vi "Open.vi"(8 "error in":errorcluster, 11 "Standard Engine in":refnum<class "Standard Engine Runtime.lvclass">) -> (0 "error out":errorcluster, 3 "Standard Engine out":refnum<class "Standard Engine Runtime.lvclass">)   [LabVIEW 2013, in "Standard Engine Runtime.lvclass"]
doc: "This VI launches an engine background process that then waits for commands from the other API functions."
uses:
  Standard Engine Runtime.lvclass
  Commands.ctl
  Engine Config Data.ctl
  Configuration/Standard Engine Configuration.lvclass
  <vilib>/NI/Tag Bus Module Framework/runtime/TBM module execution interface.lvclass
  <vilib>/NI/Tag Bus Module Framework/module configuration/TBM module configuration.lvclass
  <vilib>/NI/Module Execution Interface/Engine Runtime/Execution States.ctl
  Engine Process Init Data.ctl
  Standard Engine Runtime.lvclass/Standard Engine Runtime.ctl
  <vilib>/NI/Module Execution Interface/Engine Runtime/Engine Runtime Interface.lvclass
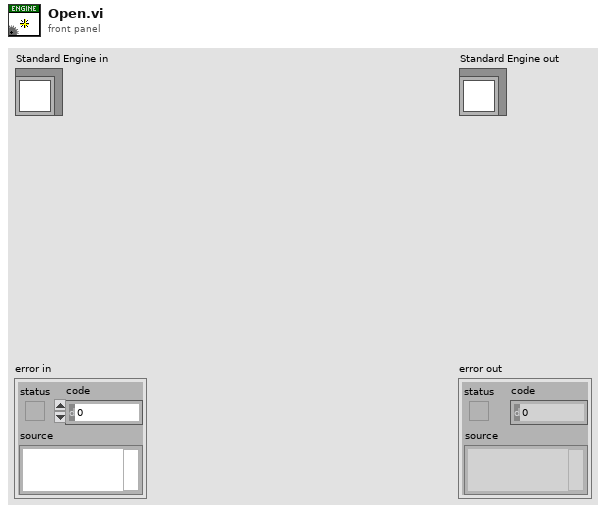
[diagram p1: front panel]
types:
  T1 = typedef "Engine Runtime Interface.lvclass/Execution States.ctl" = enum16{"Initializing", "Paused (Initialized)", "Running", "Set Safe Outputs", "Uninitializing", "Stopped (Uninitialized)", "Error (Uninitialized)", "Safe State (Uninitialized)", "Closed"}
  T2 = typedef "Standard Engine Runtime.lvclass/Engine Process Init Data.ctl" = cluster{"Messages FIFO":refnum<k33>, "Engine Config. Ref":refnum<data-value>, "Status Notifier":refnum<notifier>, "Error Queue":refnum<queue>}
  T3 = typedef "Standard Engine Runtime.lvclass/Engine Config Data.ctl" = cluster{"Engine Configuration":refnum<class "Standard Engine Configuration.lvclass">, "Modules":refnum<class "TBM module execution interface.lvclass">[], "Module Configurations":refnum<class "TBM module configuration.lvclass">[]}
  T4 = typedef "Standard Engine Runtime.lvclass/Commands.ctl" = enum16{"Initialize", "Start", "Pause", "Safe State", "Normal", "Stop", "Shutdown"}
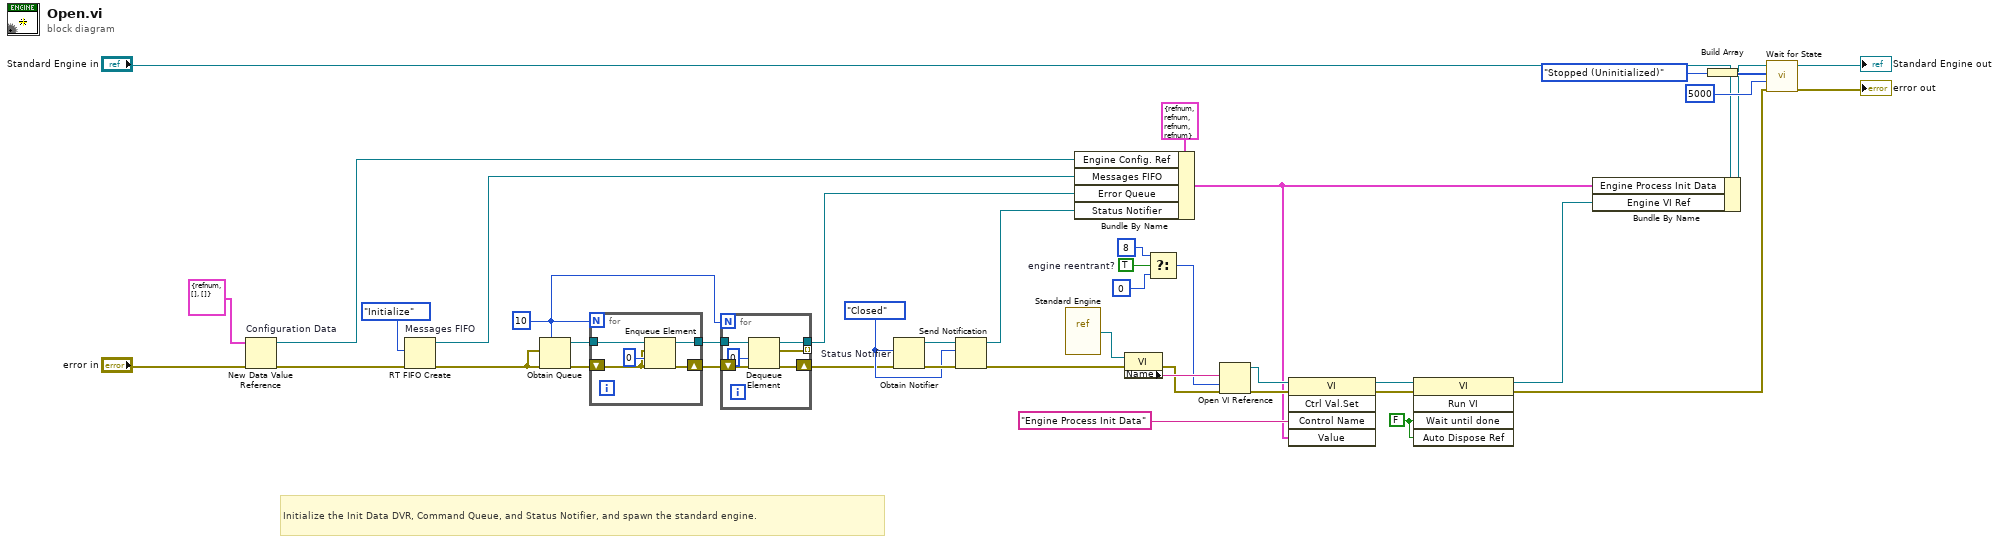
[diagram p0: block diagram]
diagram:
  w1 = FALSE ("Wait Until Done")
  w13 = TRUE  # engine reentrant?
  w23 = 10 ("max queue size (-1, unlimited)")
  w34 = Execution_States."Closed" ("States")
  # "Initialize the Init Data DVR, Command Queue, and Status Notifier, and spawn the standard engine."
  n1 = New Data Value Reference "Configuration Data"(data value=T3 {"Engine Configuration"=refnum, "Modules"=[], "Module Configurations"=[]} ("Engine Configuration Data"), error in="error in") -> (data value reference=w32:refnum<data-value>, error out=w38:errorcluster)
  n2 = RT FIFO Create "Messages FIFO"(1:Commands."Initialize" ("Commands"), 3:w38) -> (8:w31:refnum<k33>, 11:w18:errorcluster)  [unwired: 6 in, 1 out]
  n3 = Obtain Queue(max queue size (-1, unlimited)=w23, element data type=w18, error in (no error)=w18) -> (queue out=w25:refnum<queue>, error out=w24:errorcluster)  [unwired: 2 in, 1 out]
  n4 = for {
    N: w23 -> [_]
    tunnel: w25 -> [w48]
    shift-right: [w47] -> w21
    shift-left: w24 -> [w44]
    tunnel: [w45] -> w22
    n5 = Enqueue Element(queue=w48, element=w44, timeout in ms (-1)=0, error in (no error)=w44) -> (queue out=w45:refnum<queue>, error out=w47:errorcluster)  [unwired: 1 out]
  }
  n6 = for {
    N: w23 -> [_]
    tunnel: w22 -> [w54]
    shift-right: [w52] -> w19
    shift-left: w21 -> [w53]
    tunnel: [w51] -> w20
    tunnel: [w49] -> _ mode=indexing
    n7 = Dequeue Element(queue=w54, timeout in ms (-1)=0, error in (no error)=w53) -> (queue out=w51:refnum<queue>, element=w49:errorcluster, error out=w52:errorcluster)  [unwired: 1 out]
  }
  n8 = Obtain Notifier "Status Notifier"(notification data type=w34, error in (no error)=w19) -> (notifier out=w35:refnum<notifier>, error out=w36:errorcluster)  [unwired: 2 in, 1 out]
  n9 = Send Notification(notification=w34, notifier=w35, error in (no error)=w36) -> (notifier out=w30:refnum<notifier>, error out=w9:errorcluster)
  n10 = vi-ref "Standard Engine.vi"() -> (w37:refnum<vi>)
  n11 = Bundle By Name(cluster=T2 {"Messages FIFO"=refnum, "Engine Config. Ref"=refnum, "Status Notifier"=refnum, "Error Queue"=refnum} ("Engine Process Init Data"), "Engine Config. Ref"=w32, "Messages FIFO"=w31, "Error Queue"=w20, "Status Notifier"=w30) -> (w2:T2)
  n12 = property class="VI"(reference=w37, error in=w9) -> (error out=w41:errorcluster, "Name"=w42:string)  [unwired: 1 out]
  n13 = Select(t=8 ("options"), s=w13, f=0 ("options")) -> (s? t:f=w11:i32)
  n14 = Open VI Reference(vi path=w42, options=w11, error in (no error)=w41) -> (vi reference=w7:refnum<vi>, error out=w29:errorcluster)  [unwired: 3 in]
  n15 = invoke class="VI" method="Ctrl Val.Set"(reference=w7, error in=w29, "Control Name"="Engine Process Init Data", "Value"=w2) -> (reference out=w5:refnum<vi>, error out=w8:errorcluster)  [unwired: 1 in, 3 out]
  n16 = invoke class="VI" method="Run VI"(reference=w5, error in=w8, "Wait until done"=w1, "Auto Dispose Ref"=w1) -> (reference out=w4:refnum<vi>, error out=w6:errorcluster)  [unwired: 1 in, 3 out]
  n17 = Bundle By Name(cluster="Standard Engine in", "Engine Process Init Data"=w2, "Engine VI Ref"=w4) -> (w15:refnum<class "Standard Engine Runtime.lvclass">)
  n18 = Build Array(Execution_States."Stopped (Uninitialized)" ("notification")) -> (w27:T1[])
  n19 = call "Wait for State.vi"("error in"=w6, "timeout in ms"=5000, "expected states"=w27, "Standard Engine in"=w15) -> ("error out"=→"error out":errorcluster, "Standard Engine out"=→"Standard Engine out":refnum<class "Standard Engine Runtime.lvclass">)  [unwired: 6 in]
